vi "DrawScore.vi"(8 "error in (no error)":errorcluster, 10 "Game in":refnum<class "SnakeGame.lvclass">, 11 "Snake in":refnum<class "Snake.lvclass">) -> (0 "error out":errorcluster, 2 "Game out":refnum<class "SnakeGame.lvclass">, 3 "Snake out":refnum<class "Snake.lvclass">)   [LabVIEW 2019, in "RT_Game.lvlib" / "Snake.lvclass"]
uses:
  Snake.lvclass
  SnakeGame/SnakeGame.lvclass
  Snake.lvclass/Snake.ctl
  Engine/Coordinate.ctl
  Engine/Engine.lvclass
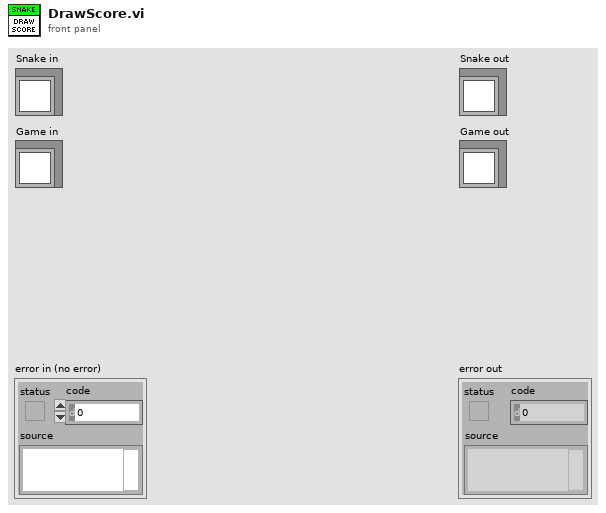
[diagram p1: front panel]
types:
  T1 = typedef "RT_Game.lvlib/Engine.lvclass/Coordinate.ctl" = cluster{"x":dbl, "y":dbl}
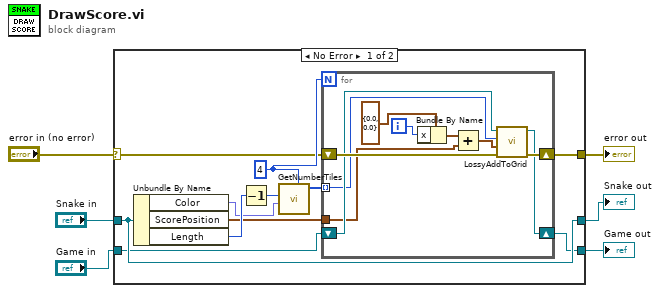
[diagram p0: block diagram]
diagram:
  n1 = case shown="No Error" "error in (no error)" {
    selector: "error in (no error)" -> [w10 w30]
    tunnel: [w9 w30] -> w5
    tunnel: [w17 w29] -> w3
    tunnel: "Snake in" -> [w17 w29]
    tunnel: [w11 w28] -> w2
    tunnel: "Game in" -> [w12 w28]
    frame No Error {
      w14 = 4 ("Digits")
      n2 = Unbundle By Name(w17) -> ("Color"=w15:fxp<+,3,3>, "ScorePosition"=w8:T1, "Length"=w16:i16)
      n3 = Decrement(x=w16) -> (x-1=w7:i16)
      n4 = call "GetNumberTiles.vi"("Digits"=w14, "Color"=w15, "score"=w7) -> ("Tiles"=w13:u32[])  [unwired: 8 in]
      n5 = for {
        N: w14 -> [_]
        tunnel: w13 -> [w23] mode=indexing
        shift-right: [w24] -> w11
        shift-left: w12 -> [w25]
        shift-right: [w26] -> w9
        shift-left: w10 -> [w27]
        tunnel: w8 -> [w22]
        i -> [w18]
        n6 = Bundle By Name(cluster=T1 {"x"=0.0, "y"=0.0} ("x"), "x"=w18) -> (w19:T1)
        n7 = Add(x=w19, y=w22) -> (x+y=w21:T1)
        n8 = call "LossyAddToGrid.vi"("error in (no error)"=w27, "Coordinate"=w21, "Tilecode"=w23, "SnakeGame in"=w25) -> ("error out"=w26:errorcluster, "SnakeGame out"=w24:refnum<class "SnakeGame.lvclass">)  [unwired: 6 in]
      }
    }
    frame Error {
    }
  }
  "error out" <- w5
  "Snake out" <- w3
  "Game out" <- w2
